vi "ARESGPS1.vi"(8 "GPS Time interval Input":dbl, 9 "Input time of last gps read":dbl, 10 "GPS Com Port":refnum<visa-resource-name>="ASRL14::INSTR", 11 "Input lat, long, dev":dbl[](array[numeric])) -> (0 "Time for GPS??":bool, 1 "Non-zero Data":bool, 2 "Zero Data":bool, 3 "Output lat, long, dev":dbl[](array[numeric]), 4 "Output time of last GPS read":dbl)   [LabVIEW 2014]
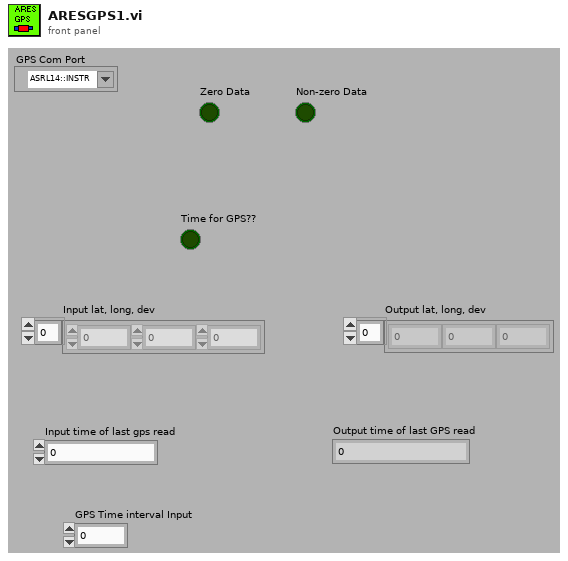
[diagram p1: front panel]
types:
  T1 = cluster{"UTC Time":timestamp, "Local Time":timestamp, "Lattitude (ddmm.mmmm)":dbl, "Lattitude North/South":string, "Longitude (ddmm.mmmm)":dbl, "Longitude East/West":string, "Magnetic Variation (degrees)":dbl, "Variation East/West":string, "Speed over ground (knots)":dbl, "Course over ground (degrees)":dbl}
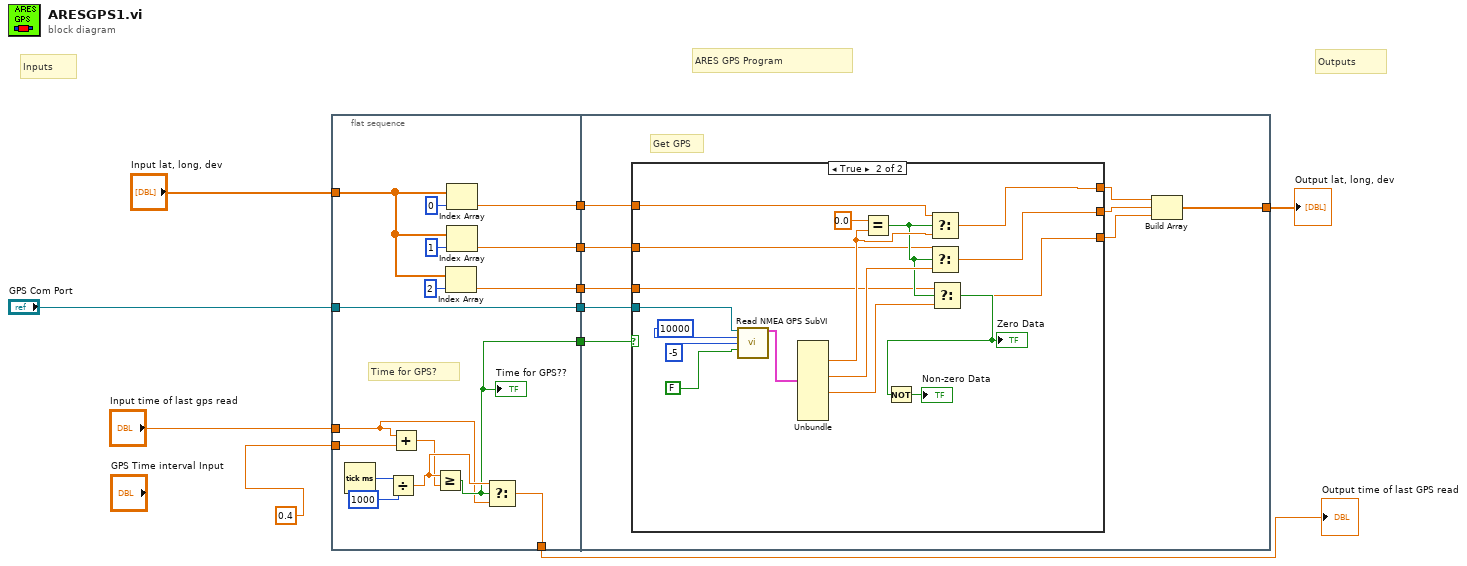
[diagram p0: block diagram]
diagram:
  # "ARES GPS Program"
  # "Outputs"
  # "Inputs"
  n1 = flat-sequence {
    tunnel: "GPS Com Port" -> [w27]
    tunnel: [w27] -> w10
    tunnel: [w22] -> w2
    tunnel: [w21] -> w9
    tunnel: "Input lat, long, dev" -> [w16]
    tunnel: [w20] -> w7
    tunnel: [w18] -> w6
    tunnel: [w14] -> w5
    tunnel: "Input time of last gps read" -> [w13]
    tunnel: 0.4 ("GPS Time interval Input") -> [w12]
    tunnel: w10 -> [w36]
    tunnel: w9 -> [w35]
    tunnel: w7 -> [w34]
    tunnel: w6 -> [w33]
    tunnel: w5 -> [w32]
    tunnel: [w28] -> w4
    frame #0 {
      # "Time for GPS?"
      n2 = Tick Count (ms)() -> (millisecond timer value=w23:u32)
      n3 = Divide(x=w23, y=u32 1000) -> (x/y=w26:dbl)
      n4 = Add(x=w13, y=w12) -> (x+y=w25:dbl)
      n5 = Greater Or Equal?(x=w26, y=w25) -> (x >= y?=w21:bool)
      "Time for GPS??" <- w21
      n6 = Index Array(array=w16, index=2) -> (element=w14:dbl)
      n7 = Index Array(array=w16, index=0) -> (element=w20:dbl)
      n8 = Index Array(array=w16, index=1) -> (element=w18:dbl)
      n9 = Select(t=w26, s=w21, f=w13) -> (s? t:f=w22:dbl)
    }
    frame #1 {
      # "Get GPS"
      n10 = case shown="True" w35 {
        tunnel: [w39 w46] -> w31
        tunnel: w36 -> [_ w45]
        tunnel: w34 -> [w39 w44]
        tunnel: w33 -> [w38 w43]
        tunnel: w32 -> [w37 w42]
        tunnel: [w37 w41] -> w29
        tunnel: [w38 w40] -> w30
        frame False {
        }
        frame True {
          n11 = call "Read NMEA GPS SubVI.vi"("VISA resource name"=w45, "timeout (ms)"=u32 10000 ("time out"), "UTC Time Zone"=-5 ("utc time zone"), "stop"=FALSE) -> ("GPS Data"=w53:T1)  [unwired: 8 in, 3 out]
          n12 = Unbundle(w53) -> ("Lattitude (ddmm.mmmm)"=w51:dbl, "Longitude (ddmm.mmmm)"=w50:dbl, "Magnetic Variation (degrees)"=w49:dbl)  [unwired: 7 out]
          n13 = Equal?(x=0.0, y=w51) -> (x = y?=w47:bool)
          "Zero Data" <- w47
          n14 = Not(x=w47) -> (.not. x?=→"Non-zero Data":bool)
          n15 = Select(t=w44, s=w47, f=w51) -> (s? t:f=w46:dbl)
          n16 = Select(t=w43, s=w47, f=w50) -> (s? t:f=w40:dbl)
          n17 = Select(t=w42, s=w47, f=w49) -> (s? t:f=w41:dbl)
        }
      }
      n18 = Build Array(w31, w30, w29) -> (w28:dbl[])
    }
  }
  "Output lat, long, dev" <- w4
  "Output time of last GPS read" <- w2
